vi "K2000_config_fastsweep.vi"(1 "error in 2":errorcluster, 2 "Readout_inst_parameters":T1, 3 "readings":u16=2 min=2 max=1024 step=1) -> (0 "error out":errorcluster)   [LabVIEW 2013]
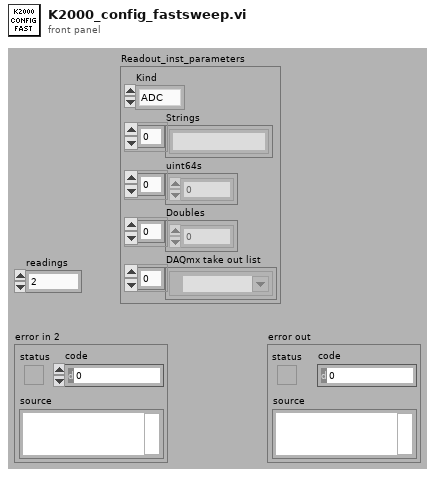
[diagram p1: front panel]
types:
  T1 = cluster{"Kind":enum16{"ADC", "K2000", "34401A", "LeCroy"}, "Strings":string[], "uint64s":u64[], "Doubles":dbl[], "DAQmx take out list":refnum<k21>[]}
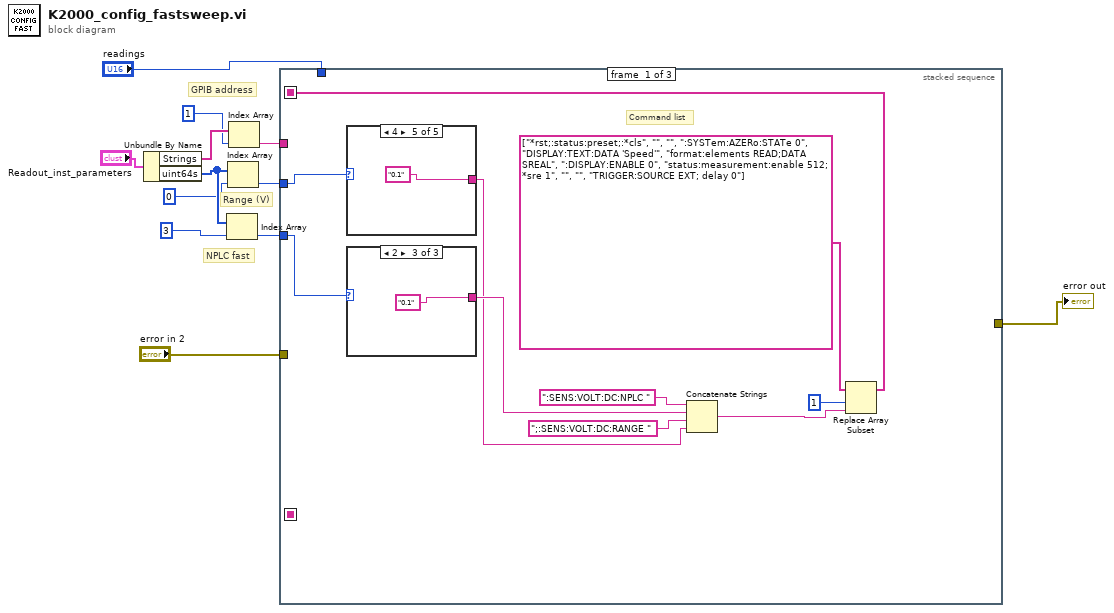
[diagram p0: block diagram]
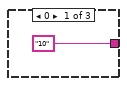
[diagram p2: hidden frame]
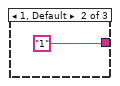
[diagram p3: hidden frame]
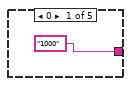
[diagram p4: hidden frame]
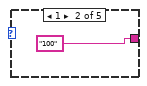
[diagram p5: hidden frame]
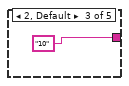
[diagram p6: hidden frame]
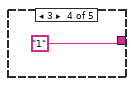
[diagram p7: hidden frame]
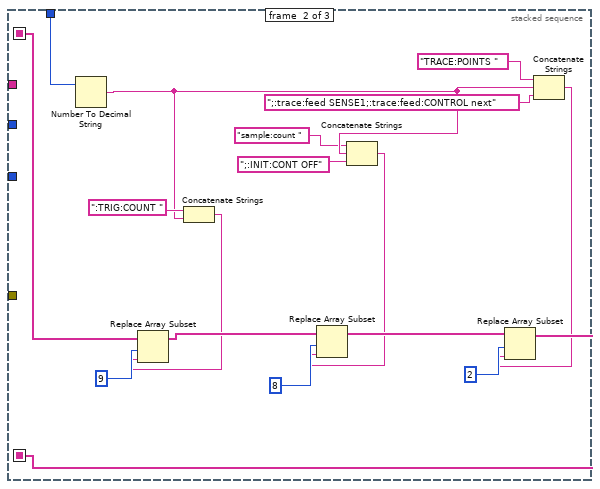
[diagram p8: hidden frame]
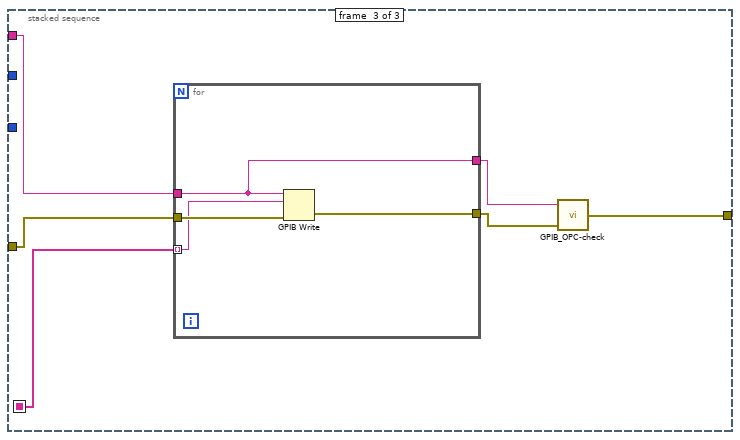
[diagram p9: hidden frame]
diagram:
  # "GPIB address"
  # "Range (V)"
  # "NPLC fast"
  n1 = Unbundle By Name("Readout_inst_parameters") -> ("Strings"=w11:string[], "uint64s"=w10:u64[])
  n2 = Index Array(array=w10, index=3) -> (element=w4:u64)
  n3 = Index Array(array=w10, index=0) -> (element=w5:u64)
  n4 = Index Array(array=w11, index=1) -> (element=w6:string)
  n5 = stacked-sequence {
    seq-local: [w13 _ _] -> [_ w39 _]
    seq-local: [_ w36 _] -> [_ _ w48]
    tunnel: w6 -> [_ _ w53]
    tunnel: w5 -> [w22 _ _]
    tunnel: w4 -> [w21 _ _]
    tunnel: "readings" -> [_ w47 _]
    tunnel: "error in 2" -> [_ _ w52]
    tunnel: [_ _ w49] -> w1
    frame #0 {
      # "Command list"
      n6 = case shown="4" w22 {
        tunnel: ["1000" "100" "10" "1" "0.1"] -> w17
        frame 0 {
        }
        frame 1 {
        }
        frame 2, Default {
        }
        frame 3 {
        }
        frame 4 {
        }
      }
      n7 = case shown="2" w21 {
        tunnel: ["10" "1" "0.1"] -> w18
        frame 0 {
        }
        frame 1, Default {
        }
        frame 2 {
        }
      }
      n8 = Concatenate Strings(":SENS:VOLT:DC:NPLC " ("string"), w18, ";:SENS:VOLT:DC:RANGE " ("string"), w17) -> (w14:string)
      n9 = Replace Array Subset(array=string[] ["*rst;:status:preset;:*cls", "", "", ":SYSTem:AZERo:STATe 0", "DISPLAY:TEXT:DATA 'Speed'", "format:elements READ;DATA SREAL", ":DISPLAY:ENABLE 0", "status:measurement:enable 512; *sre 1", "", "", "TRIGGER:SOURCE EXT; delay 0"], new element=w14, index=1) -> (w13:string[])
    }
    frame #1 {
      n10 = Number To Decimal String(number=w47) -> (decimal integer string=w43:string)  [unwired: 1 in]
      n11 = Concatenate Strings(":TRIG:COUNT " ("data"), w43) -> (w33:string)
      n12 = Replace Array Subset(array=w39, new element=w33, index=9) -> (w38:string[])
      n13 = Concatenate Strings("sample:count " ("data"), w43, ";:INIT:CONT OFF" ("string")) -> (w32:string)
      n14 = Replace Array Subset(array=w38, new element=w32, index=8) -> (w37:string[])
      n15 = Concatenate Strings("TRACE:POINTS " ("data"), w43, ";:trace:feed SENSE1;:trace:feed:CONTROL next" ("string")) -> (w31:string)
      n16 = Replace Array Subset(array=w37, new element=w31, index=2) -> (w36:string[])
    }
    frame #2 {
      n17 = for {
        tunnel: w53 -> [w55]
        tunnel: w52 -> [w57]
        tunnel: [w56] -> w50
        tunnel: [w55] -> w51
        tunnel: w48 -> [w54] mode=indexing
        n18 = GPIB Write(0:w55, 1:w54, 3:w57) -> (6:w56:errorcluster)  [unwired: 3 out]
      }
      n19 = call "GPIB_OPC-check.vi"("error out 2"=w50, "GPIB Address"=w51) -> ("error out"=w49:errorcluster)  [unwired: 1 out]
    }
  }
  "error out" <- w1
